vi "RecoverFromIronsSuggestion.vi"(6 "Old Suggested Sail Setpoints":T1 {"MainSailSuggestion" min=0.0 max=1.0; "JibSailSuggestion" min=0.0 max=1.0}, 9 "RelativeWindAngle":dbl, 10 "DesiredHeading":dbl, 11 "RobotHeading":dbl) -> (2 "Suggested Rudder Set Point":dbl, 3 "Suggested Sail Setpoints":T1 {"MainSailSuggestion" min=0.0 max=1.0; "JibSailSuggestion" min=0.0 max=1.0})   [LabVIEW 2012]
doc: "Set the sails and rudder in such a way as to help the boat recover from irons.\n\nRelevant when heading matches wind direction within some range.\n\n3 proposed modes:\n\"Helpless\" waits for a wind change to turn the boat, pulls the sails in.\n(Maybe the jib more than the main to try to get more torque on the front?)\n\"Recovering\" once turn is sensed throws the rudder into the direction of turn to generate some additional angular momentum in that direction.\n\"Sculling\" tries to use the rudder to get out of a helpless mode.\n\nMichael Bocamazo Jan 2014"
uses:
  Data/TypeDefs/Sail Set Suggestions.ctl
panel:
  # "Sets the sails in such a way as to help the boat turn\nin the desired direction. Turning upwind, for example,\nwould involve overpowering the main and underpowering\nthe jib.\n\nWhen exactly this setting should be used is unclear, it\nprobably shouldn't be used for small turns until much testing\nhas been done to make sure it doesn't interfere with regular\nsail operations. At the moment it seems reasonable to use\nthis to help the boat turn large angles at low speeds. At higher\nspeeds the rudder should be effective to turn the boat.\n\nSuggestion: ONLY calculate how to set the sails to help\nturn the boat in this VI, use the arbiter to decide when\nto use the sails to turn."
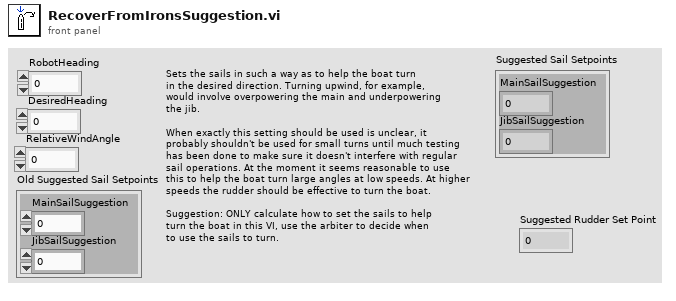
[diagram p1: front panel]
types:
  T1 = typedef "Sail Set Suggestions.ctl" = cluster{"MainSailSuggestion":dbl, "JibSailSuggestion":dbl}
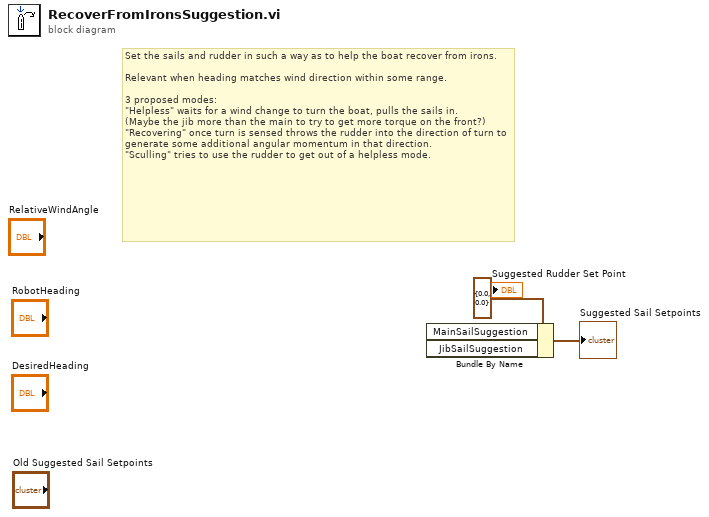
[diagram p0: block diagram]
diagram:
  # "Set the sails and rudder in such a way as to help the boat recover from irons.\n\nRelevant when heading matches wind direction within some range.\n\n3 proposed modes:\n\"Helpless\" waits for a wind change to turn the boat, pulls the sails in.\n(Maybe the jib more than the main to try to get more torque on the front?)\n\"Recovering\" once turn is sensed throws the rudder into the direction of turn to generate some additional angular momentum in that direction.\n\"Sculling\" tries to use the rudder to get out of a helpless mode."
  n1 = Bundle By Name(cluster=T1 {"MainSailSuggestion"=0.0, "JibSailSuggestion"=0.0} ("output cluster")) -> (→"Suggested Sail Setpoints":T1)  [unwired: 2 in]
